vi "Gobal for ROS.vi"() -> ()   [LabVIEW 2015]
panel:
  in  "String 2":string="GET / HTTP/1.1\nUpgrade: websocket\nConnection: Upgrade\nHost: 192.168.212.128:9090\nSec-WebSocket-Key: pM4mFvl5nUXJXjxIa41LvQ==\nSec-WebSocket-Version: 13\n\n"
  in  "STEERING":T1
  in  "szablon CMD_VEL":T2
  in  "String":string="GET / HTTP/1.1\nUpgrade: websocket\nConnection: Upgrade\nHost: 192.168.5.103:9090\nOrigin: http://192.168.5.101:9090\nSec-WebSocket-Key: pM4mFvl5nUXJXjxIa41LvQ==\nSec-WebSocket-Version: 13"
  in  "rosbridge port":u16=9090
  in  "rosbridge server IP":string="192.168.1.117"
  out "ROS read":T3
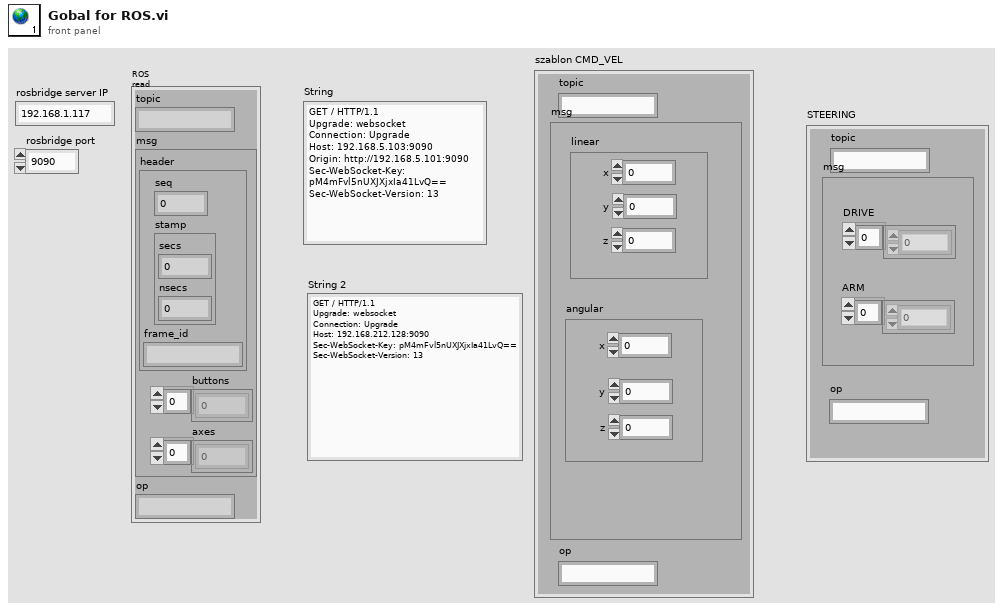
[diagram p1: front panel]
types:
  T1 = cluster{"topic":string, "msg":cluster{"DRIVE":i16[], "ARM":i8[]}, "op":string}
  T2 = cluster{"topic":string, "msg":cluster{"linear":cluster{"x":dbl, "y":dbl, "z":dbl}, "angular":cluster{"x":dbl, "y":dbl, "z":dbl}}, "op":string}
  T3 = cluster{"topic":string, "msg":cluster{"header":cluster{"seq":u32, "stamp":cluster{"secs":u32, "nsecs":i32}, "frame_id":string}, "buttons":i32[], "axes":sgl[]}, "op":string}
diagram:
